vi "PC new main.vi"() -> ()   [LabVIEW 2020]
uses:
  <vilib>/FPGAPlugInAG/PXI-7951R/niLvFpga_Open_PXI-7951R.vi
  <vilib>/rvi/interface/common/dynamic/niFpgaDynamicAddResources.vi
  <vilib>/FPGAPlugInAG/Dynamic/niLvFpga_Abort_Dynamic.vi
  <vilib>/rvi/interface/common/niFpgaWaitOnOcc.vi
  <vilib>/Utility/error.llb/Error Cluster From Error Code.vi
  <vilib>/FPGAPlugInAG/Dynamic/niLvFpga_Run_Dynamic.vi
  <vilib>/LabVIEW Targets/FPGA/FlexRIO/CustomFPGAMethods/79XXR_Method_IOModuleStatusImpl.vi
  <vilib>/rvi/errors/niLvFpgaAdjustHostInterfaceError.vi
  <vilib>/FPGAPlugInAG/Dynamic/niLvFpga_Close_Dynamic.vi
  <vilib>/rvi/interface/nirviOpenFPGA/nirviOpenFPGA.xnode
  FPGA Bitfiles/juanmultiple_FPGATarget_FPGAnewmain_DGOcCx6UUYc.lvbitx
  <vilib>/rvi/interface/nirviMethod/nirviMethod.xnode
  <vilib>/rvi/interface/nirviReadWriteControl/nirviReadWriteControl.xnode
  <vilib>/rvi/interface/nirviCloseFPGA/nirviCloseFPGA.xnode
  <vilib>/rvi/errors/niLvFpgaMergeErrorWithErrorCode.vi
  <vilib>/FPGAPlugInAG/Dynamic/niLvFpga_ReadFifo_Dynamic.vi
  <vilib>/rvi/interface/Simulation/niFpgaSimulationCallBeginRW.vi
  <vilib>/FPGAPlugInAG/Dynamic/niLvFpga_ConfigureFifo_Dynamic.vi
  NiFpgaLv.dll
panel:
  out "binary error status":errorcluster
  in  "Iter per file":i32
  out "current iter":i32
  out "Elements Remaining":u32
  out "running time (s)":dbl
  in  "max iter":i32
  out "daq status":errorcluster
  out "Actual Depth":u32
  in  "Requested Depth":u32
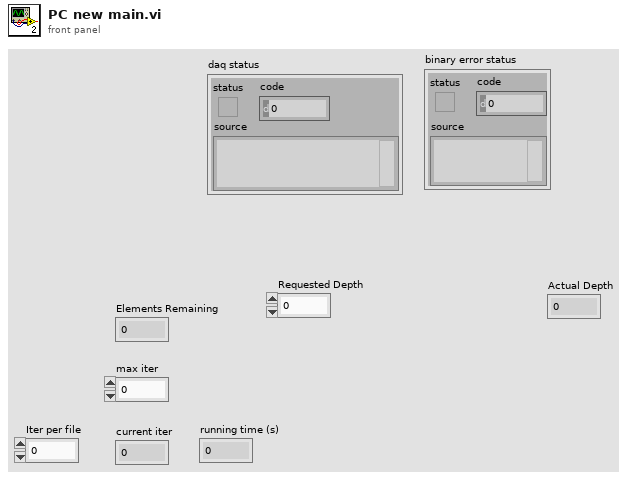
[diagram p1: front panel]
types:
  T1 = enum16{"open", "replace", "create", "open or create", "replace or create", "replace or create with confirmation"}
  T2 = enum16{"big-endian, network order", "native, host order", "little-endian"}
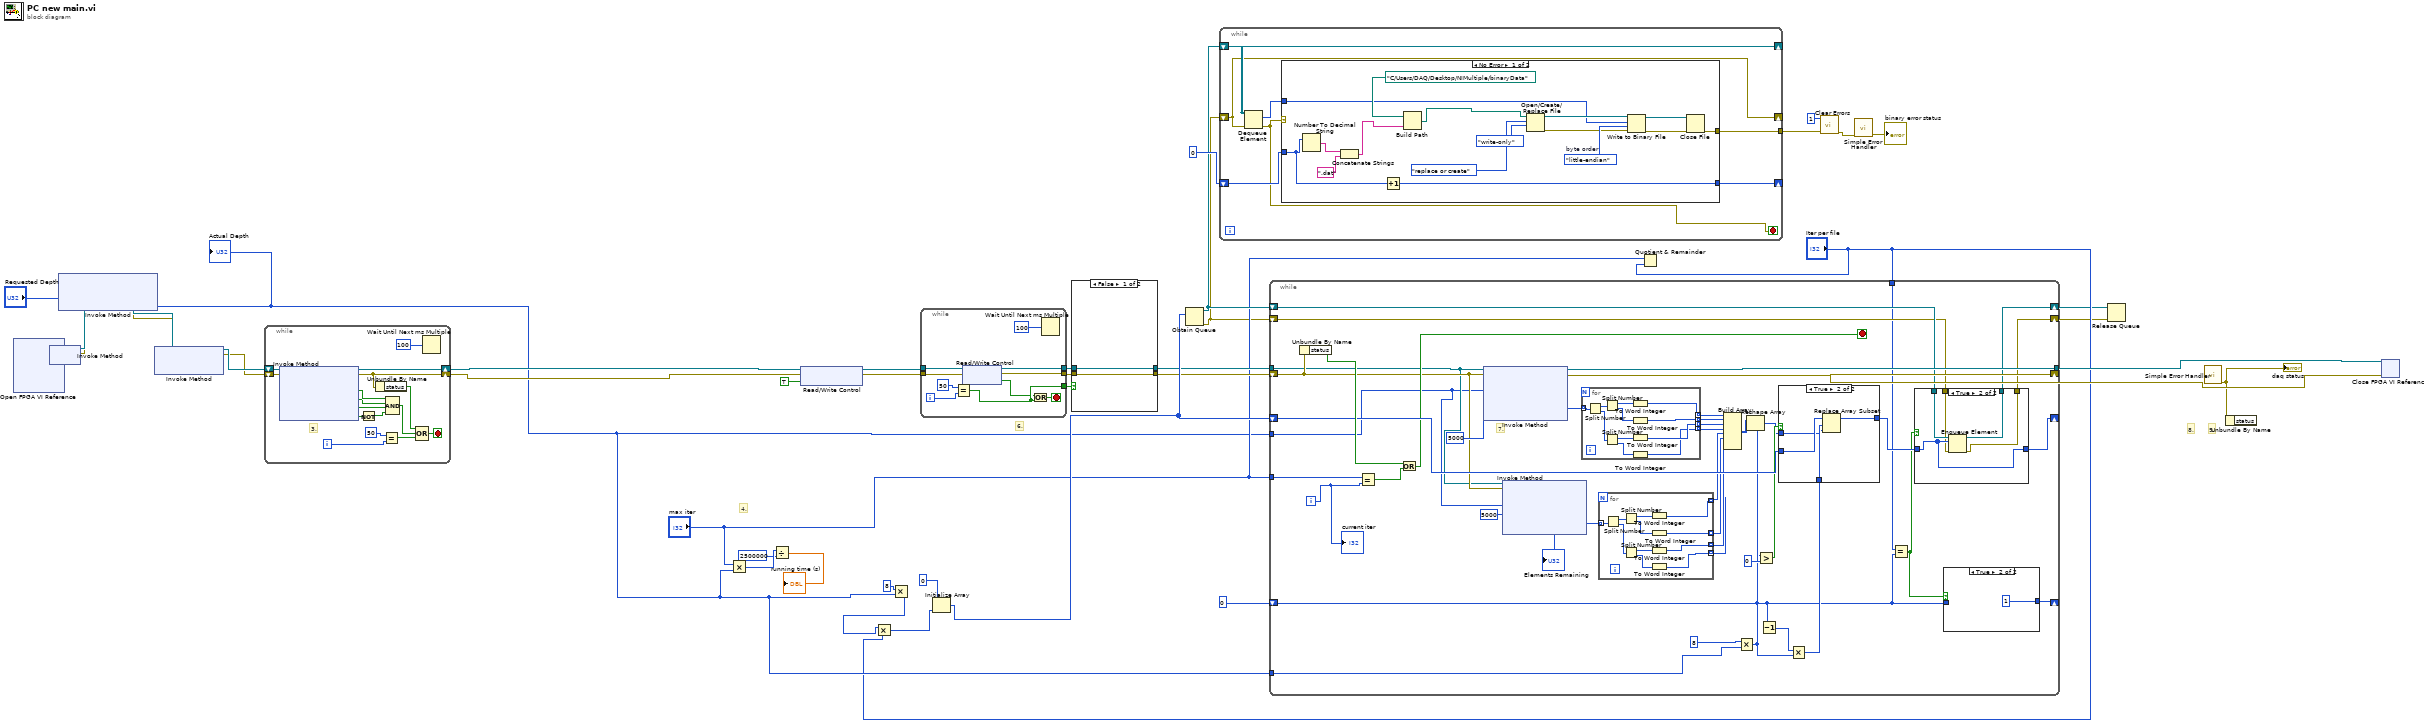
[diagram p0: block diagram]
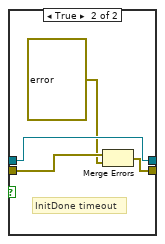
[diagram p2: hidden frame]
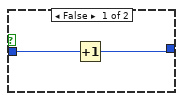
[diagram p3: hidden frame]
diagram:
  # "6."
  # "4."
  # "9."
  # "8."
  n1 = xnode "Open FPGA VI Reference"() -> ("FPGA VI Reference Out"=w41:refnum<k20>, "error out"=w40:errorcluster)  [unwired: 2 in]
  n2 = xnode "Invoke Method"("FPGA VI Reference In"=w41, "error in"=w40) -> ("FPGA VI Reference Out"=w35:refnum<k20>, "error out"=w33:errorcluster)
  n3 = xnode "Invoke Method"("FPGA VI Reference In"=w35, "error in"=w33, "Requested Depth"="Requested Depth") -> ("FPGA VI Reference Out"=w34:refnum<k20>, "error out"=w32:errorcluster, "Actual Depth"=w8:u32)
  "Actual Depth" <- w8
  n4 = xnode "Invoke Method"("FPGA VI Reference In"=w34, "error in"=w32) -> ("FPGA VI Reference Out"=w37:refnum<k20>, "error out"=w36:errorcluster)  [unwired: 1 in]
  n5 = while {
    shift-right: [w50] -> w39
    shift-left: w36 -> [w58]
    shift-right: [w57] -> w38
    shift-left: w37 -> [w59]
    i -> [w52]
    stop <- w47 stop-if-true
    # "3."
    n6 = xnode "Invoke Method"("FPGA VI Reference In"=w59, "error in"=w58) -> ("FPGA VI Reference Out"=w57:refnum<k20>, "error out"=w50:errorcluster, "IO Module Present?"=w56:bool, "Power Enabled?"=w55:bool, "IO Enabled?"=w54:bool, "IO Module Mismatch?"=w45:bool)
    n7 = Not(x=w45) -> (.not. x?=w44:bool)
    n8 = Unbundle By Name(w50) -> ("status"=w49:bool)
    n9 = Equal?(x=50, y=w52) -> (x = y?=w46:bool)
    n10 = Compound Arithmetic op=AND(w56, w55, w54, w44) -> (w48:bool)
    n11 = Compound Arithmetic op=OR(w49, w48, w46) -> (w47:bool)
    n12 = Wait Until Next ms Multiple(millisecond multiple=u32 100) -> ()  [unwired: 1 out]
  }
  n13 = Multiply(x="max iter", y=w8) -> (x*y=w25:u32)
  n14 = Divide(x=w25, y=2500000) -> (x/y=→"running time (s)":dbl)
  n15 = xnode "Read/Write Control"("FPGA VI Reference In"=w38, "error in"=w39, "Start Acquisition"=TRUE) -> ("FPGA VI Reference Out"=w16:refnum<k20>, "error out"=w17:errorcluster)
  n16 = Multiply(x=8, y=w8) -> (x*y=w7:u32)
  n17 = Multiply(x=w7, y="Iter per file") -> (x*y=w26:u32)
  n18 = while {
    tunnel: w16 -> [w69]
    tunnel: [w65] -> w19
    tunnel: [w64] -> w18
    tunnel: [w62] -> w20
    tunnel: w17 -> [w60]
    i -> [w67]
    stop <- w63 stop-if-true
    n19 = Equal?(x=50, y=w67) -> (x = y?=w62:bool)
    n20 = xnode "Read/Write Control"("FPGA VI Reference In"=w69, "error in"=w60) -> ("FPGA VI Reference Out"=w65:refnum<k20>, "error out"=w64:errorcluster, "Init Done"=w61:bool)
    n21 = Or(x=w61, y=w62) -> (x .or. y?=w63:bool)
    n22 = Wait Until Next ms Multiple(millisecond multiple=u32 100) -> ()  [unwired: 1 out]
  }
  n23 = Initialize Array(i16 0 ("element"), w26) -> (w28:i16[])
  n24 = case shown="False" w20 {
    tunnel: [w71 w75] -> w15
    tunnel: w19 -> [w71 w75]
    tunnel: w18 -> [w70 w73]
    tunnel: [w70 w74] -> w14
    frame False {
    }
    frame True {
      # "InitDone timeout"
      n25 = Merge Errors(w73, errorcluster {"status"=TRUE, "code"=-1, "source"="The IO Module CLIP was not ready. If you are using any external clocks, make sure they are connected and within the supported specifications."} ("error in")) -> (w74:errorcluster)
    }
  }
  n26 = Obtain Queue(element data type=w28) -> (queue out=w12:refnum<queue>, error out=w9:errorcluster)  [unwired: 4 in, 1 out]
  n27 = while {
    tunnel: [w82] -> w3
    shift-right: [w80] -> _
    shift-left: 0 -> [w77]
    shift-right: [w79] -> _
    shift-left: w12 -> [w79]
    shift-right: [w78] -> _
    shift-left: w9 -> [w78]
    stop <- w76 stop-if-true
    n28 = Dequeue Element(queue=w79, error in (no error)=w78) -> (element=w81:i16[], error out=w76:errorcluster)  [unwired: 1 in, 2 out]
    n29 = case shown="No Error" w76 {
      selector: w76 -> [_ w99]
      tunnel: [w93 w99] -> w82
      tunnel: w81 -> [w89 _]
      tunnel: w77 -> [w85 w100]
      tunnel: [w84 w100] -> w80
      frame No Error {
        w92 = T2."little-endian"  # byte order
        n30 = Number To Decimal String(number=w85) -> (decimal integer string=w87:string)  [unwired: 1 in]
        n31 = Concatenate Strings(w87, ".dat" ("string")) -> (w86:string)
        n32 = Increment(x=w85) -> (x+1=w84:i32)
        n33 = Build Path(base path=path "C:/Users/DAQ/Desktop/NIMultiple/binaryData", name or relative path=w86) -> (appended path=w83:path)
        n34 = Open/Create/Replace File(file path (use dialog)=w83, operation (0:open)=T1."replace or create", access (0:read/write)=enum16{"read/write", "read-only", "write-only"}."write-only") -> (refnum out=w91:refnum<file>, error out=w90:errorcluster)  [unwired: 3 in, 1 out]
        n35 = Write to Binary File(file (use dialog)=w91, data=w89, error in=w90, 9:w92) -> (refnum out=w98:refnum<file>, error out=w97:errorcluster)  [unwired: 2 in, 1 out]
        n36 = Close File(refnum=w98, error in=w97) -> (error out=w93:errorcluster)  [unwired: 1 out]
      }
      frame Error {
      }
    }
  }
  n37 = while {
    tunnel: [w143] -> w43
    tunnel: w15 -> [w102]
    shift-right: [w142] -> w42
    shift-left: w14 -> [w103]
    tunnel: w8 -> [w101]
    tunnel: "max iter" -> [w131]
    shift-right: [w115] -> _
    shift-left: w28 -> [w133]
    shift-right: [w109] -> _
    shift-left: 0 ("x") -> [w108]
    tunnel: "Iter per file" -> [w107]
    shift-right: [w106] -> w5
    shift-left: w12 -> [w113]
    shift-right: [w105] -> w4
    shift-left: w9 -> [w112]
    tunnel: w8 -> [w104]
    i -> [w111]
    stop <- w132 stop-if-true
    # "7."
    n38 = Unbundle By Name(w103) -> ("status"=w140:bool)
    n39 = Equal?(x=w131, y=w111) -> (x = y?=w141:bool)
    n40 = Or(x=w140, y=w141) -> (x .or. y?=w132:bool)
    n41 = xnode "Invoke Method"("FPGA VI Reference In"=w102, "error in"=w103, "Number of Elements"=w101, "Timeout (ms)"=5000) -> ("FPGA VI Reference Out"=w143:refnum<k20>, "error out"=w142:errorcluster, "Data"=w138:i16[])  [unwired: 1 out]
    n42 = xnode "Invoke Method"("FPGA VI Reference In"=w102, "error in"=w103, "Number of Elements"=w101, "Timeout (ms)"=5000) -> ("Data"=w136:u16[], "Elements Remaining"=→"Elements Remaining":u32)  [unwired: 2 out]
    n43 = for {
      tunnel: w138 -> [w159] mode=indexing
      tunnel: [w158] -> w124 mode=indexing
      tunnel: [w157] -> w123 mode=indexing
      tunnel: [w156] -> w122 mode=indexing
      tunnel: [w155] -> w121 mode=indexing
      n44 = Split Number(x=w159) -> (hi(x)=w165:u8, lo(x)=w164:u8)
      n45 = Split Number(x=w165) -> (hi(x)=w163:u8, lo(x)=w162:u8)
      n46 = Split Number(x=w164) -> (hi(x)=w161:u8, lo(x)=w160:u8)
      n47 = To Word Integer(number=w163) -> (16bit integer=w158:i16)
      n48 = To Word Integer(number=w162) -> (16bit integer=w157:i16)
      n49 = To Word Integer(number=w161) -> (16bit integer=w156:i16)
      n50 = To Word Integer(number=w160) -> (16bit integer=w155:i16)
    }
    n51 = for {
      tunnel: w136 -> [w148] mode=indexing
      tunnel: [w147] -> w120 mode=indexing
      tunnel: [w146] -> w119 mode=indexing
      tunnel: [w145] -> w118 mode=indexing
      tunnel: [w144] -> w117 mode=indexing
      n52 = Split Number(x=w148) -> (hi(x)=w154:u8, lo(x)=w153:u8)
      n53 = Split Number(x=w154) -> (hi(x)=w152:u8, lo(x)=w151:u8)
      n54 = Split Number(x=w153) -> (hi(x)=w150:u8, lo(x)=w149:u8)
      n55 = To Word Integer(number=w152) -> (16bit integer=w147:i16)
      n56 = To Word Integer(number=w151) -> (16bit integer=w146:i16)
      n57 = To Word Integer(number=w150) -> (16bit integer=w145:i16)
      n58 = To Word Integer(number=w149) -> (16bit integer=w144:i16)
    }
    n59 = Build Array(w124, w123, w122, w121, w120, w119, w118, w117) -> (w127:i16[][])
    n60 = Multiply(x=8, y=w104) -> (x*y=w116:u32)
    n61 = Reshape Array(w127, w116) -> (w125:i16[])
    n62 = Greater?(x=w108, y=0) -> (0:w130:bool)
    n63 = Decrement(x=w108) -> (x-1=w128:i32)
    n64 = Multiply(x=w128, y=w116) -> (x*y=w129:u32)
    n65 = case shown="True" w130 {
      tunnel: w133 -> [w177 w181]
      tunnel: [w177 w180] -> w114
      tunnel: w129 -> [_ w179]
      tunnel: w125 -> [_ w178]
      frame False {
      }
      frame True {
        n66 = Replace Array Subset(array=w181, new element=w178, index=w179) -> (w180:i16[])
      }
    }
    n67 = Equal?(x=w107, y=w108) -> (x = y?=w110:bool)
    n68 = case shown="True" w110 {
      tunnel: [w171 w176] -> w115
      tunnel: w114 -> [w171 w176]
      tunnel: w113 -> [w169 w175]
      tunnel: w112 -> [w170 w174]
      tunnel: [w169 w173] -> w106
      tunnel: [w170 w172] -> w105
      frame False {
      }
      frame True {
        n69 = Enqueue Element(queue=w175, element=w176, error in (no error)=w174) -> (queue out=w173:refnum<queue>, error out=w172:errorcluster)  [unwired: 1 in, 1 out]
      }
    }
    n70 = case shown="True" w110 {
      tunnel: [w166 1 ("y")] -> w109
      tunnel: w108 -> [w167 _]
      frame False {
        n71 = Increment(x=w167) -> (x+1=w166:i32)
      }
      frame True {
      }
    }
    "current iter" <- w111
  }
  n72 = Quotient & Remainder(x="max iter", y="Iter per file") -> ()  [unwired: 2 out]
  n73 = call <vilib>:"Clear Errors.vi"("error in (no error)"=w3, "specific error code to clear (0: all)"=1) -> ("error out"=w2:errorcluster)  [unwired: 4 in, 1 out]
  n74 = call <vilib>:"Simple Error Handler.vi"("error in (no error)"=w2) -> ("error out"=→"binary error status":errorcluster)  [unwired: 1 in, 7 out]
  n75 = Release Queue(queue=w5, error in (no error)=w4) -> ()  [unwired: 1 in, 3 out]
  n76 = call <vilib>:"Simple Error Handler.vi"() -> ("error out"=w30:errorcluster)  [unwired: 2 in, 7 out]
  "daq status" <- w30
  n77 = Unbundle By Name(w30) -> ()  [unwired: 1 out]
  n78 = xnode "Close FPGA VI Reference"("FPGA VI Reference In"=w43, "error in"=w42) -> ()  [unwired: 1 out]
